vi "XPath表达式.vi"(7 "添加的路径":path, 11 "XPath expression":string caption="XPath表达式") -> (3 "数组":string[](array[string]))   [LabVIEW 2016, in "斯坦道CODcr.lvlib"]
uses:
  <vilib>/xml/Load XML File.vi
  <vilib>/xml/Close Reference(Node).vi
  <vilib>/xml/NI_XML.lvlib
  <resource>/objmgr/DOMUserDefRef.rc
panel:
  out "XML字符串":string="<?xml version=\"1.0\" encoding=\"ISO-8859-1\"?>\n<bookstore>\n<book ISBN=\"978-0545128285\">\n  <title lang=\"en\">The Tales of Beedle the Bard</title>\n  <author>J. K. Rowling</author>\n  <year>2008</year>\n  <price>12.99</price>\n</book>\n<book ISBN=\"978-0316160209\">\n  <title lang=\"en\">Eclipse</title>\n  <author>Stephenie Meyer</author>\n  <year>2007</year>\n  <price>19.99</price>\n</book>\n<book ISBN=\"978-0316067928\">\n  <title lang=\"en\">Breaking Dawn</title>\n  <author>Stephenie Meyer</author>\n  <year>2008</year>\n  <price>22.99</price>\n</book>\n<book ISBN=\"978-0316017923\">\n  <title lang=\"en\">Outliers: The Story of Success</title>\n  <author>Malcolm Gladwell</author>\n  <year>2008</year>\n  <price>27.99</price>\n</book>\n<book ISBN=\"978-0596007645\">\n  <title lang=\"en\">XML in a Nutshell</title>\n  <author>Elliotte Rusty Harold</author>\n  <author>W. Scott Means</author>\n  <year>2004</year>\n  <price>39.95</price>\n</book>\n</bookstore>"
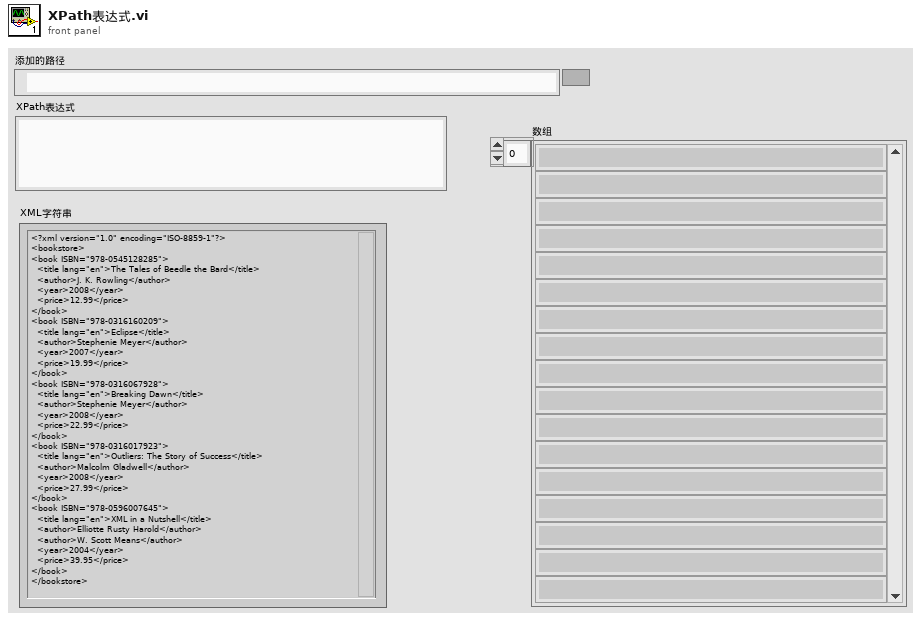
[diagram p1: front panel]
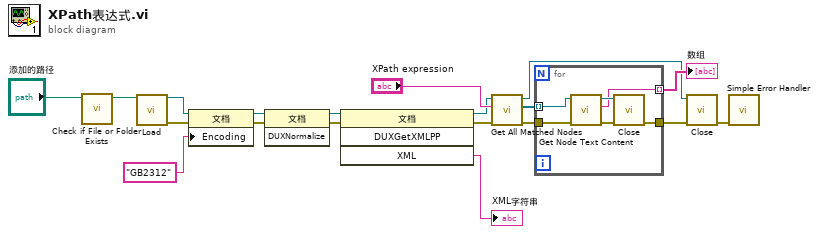
[diagram p0: block diagram]
diagram:
  n1 = call <vilib>:"Check if File or Folder Exists.vi"("path"="添加的路径") -> ("dup path"=w18:path)  [unwired: 8 in, 2 out]
  n2 = call-poly <vilib>:"Load.vi"("path to XML document"=w18) -> ("DOM document out"=w15:refnum<k20>, "error out"=w14:errorcluster)  [unwired: 12 in, 1 out]
  n3 = property on="属性节点" class="文档"(reference=w15, error in=w14, "Encoding"="GB2312" ("文档编码")) -> (reference out=w13:refnum<k20>, error out=w12:errorcluster)
  n4 = invoke on="Invoke Node" class="文档" method="DUXNormalize"(reference=w13, error in=w12) -> (reference out=w10:refnum<k20>, error out=w11:errorcluster)  [unwired: 1 in, 1 out]
  n5 = invoke on="Invoke Node" class="文档" method="DUXGetXMLPP"(reference=w10, error in=w11) -> (reference out=w1:refnum<k20>, error out=w2:errorcluster, "XML"=→"XML字符串":string)  [unwired: 2 in, 1 out]
  n6 = call <vilib>:"Get All Matched Nodes.vi"("error in (no error)"=w2, "XPath expression"="XPath expression", "node in"=w1) -> ("error out"=w7:errorcluster, "node result array"=w8:refnum<k20>[], "node out"=w4:refnum<k20>)  [unwired: 6 in]
  n7 = for {
    tunnel: w7 -> [w25]
    tunnel: [w22] -> w5 mode=indexing
    tunnel: w8 -> [w20] mode=indexing
    tunnel: [w21] -> w3
    n8 = call <vilib>:"Get Node Text Content.vi"("error in (no error)"=w25, "node in"=w20) -> ("error out"=w23:errorcluster, "node text"=w22:string, "node out"=w24:refnum<k20>)  [unwired: 7 in]
    n9 = call-poly <vilib>:"Close.vi"("error in (no error)"=w23, "node"=w24) -> ("error out"=w21:errorcluster)  [unwired: 7 out]
  }
  "数组" <- w5
  n10 = call-poly <vilib>:"Close.vi"("error in (no error)"=w3, "node"=w4) -> ("error out"=w17:errorcluster)  [unwired: 7 out]
  n11 = call <vilib>:"Simple Error Handler.vi"("error in (no error)"=w17) -> ()  [unwired: 4 in, 5 out]
